vi "New Array.vi"(7 "prev index":i32, 8 "new index":i32, 9 "Array":T1[](array[typedef]), 10 "prev element":cluster{"X":dbl, "Y":dbl, "Z":dbl}, 11 "array":T2) -> (3 "array out":T2)   [LabVIEW 2014]
uses:
  Libraries/Map Data Folder/All-Lines.ctl
  Libraries/Map Data Folder/LineCluster.ctl
  Libraries/Map Data Folder/LineConnection.ctl
  Libraries/Contact Data/Position.ctl
  Libraries/Map Data Folder/Map Data.lvlib
  Libraries/Contact Data/Contact Data.lvlib
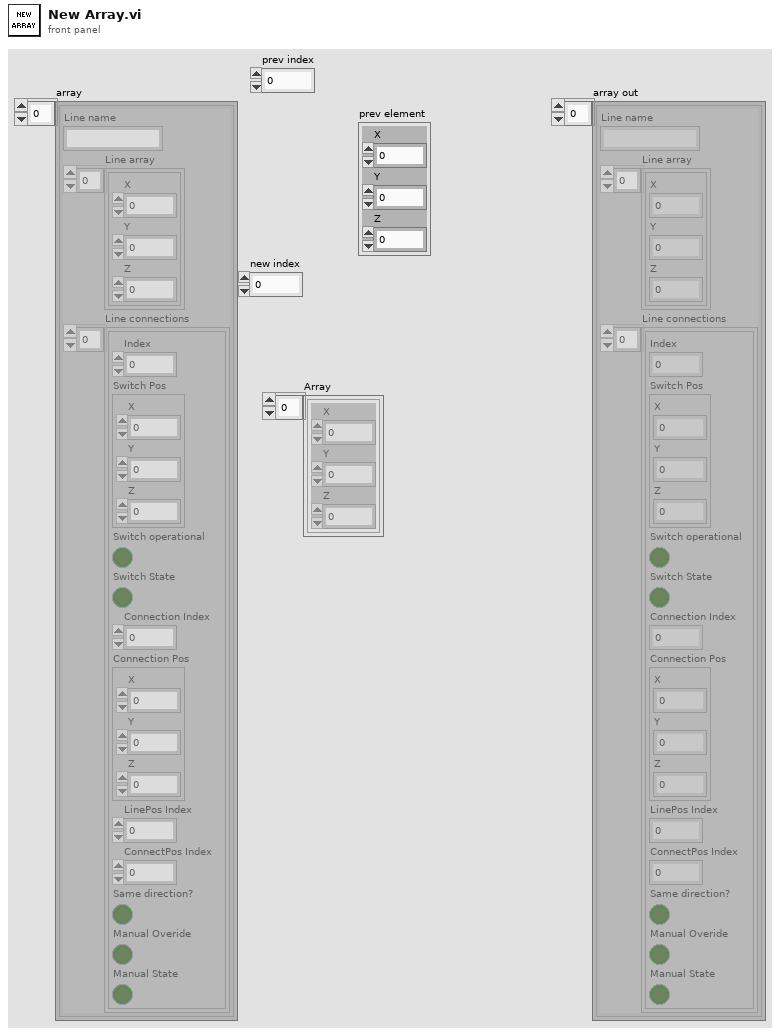
[diagram p1: front panel]
types:
  T1 = typedef "Contact Data.lvlib/Position.ctl" = cluster{"X":dbl, "Y":dbl, "Z":dbl}
  T2 = typedef "Map Data.lvlib/All-Lines.ctl" = T3[]
  T3 = typedef "Map Data.lvlib/LineCluster.ctl" = cluster{"Line name":string, "Line array":cluster{"X":dbl, "Y":dbl, "Z":dbl}[], "Line connections":T4[]}
  T4 = typedef "LineConnection.ctl" = cluster{"Index":i32, "Switch Pos":cluster{"X":dbl, "Y":dbl, "Z":dbl}, "Switch operational":bool, "Switch State":bool, "Connection Index":i32, "Connection Pos":cluster{"X":dbl, "Y":dbl, "Z":dbl}, "LinePos Index":i32, "ConnectPos Index":i32, "Same direction?":bool, "Manual Overide":bool, "Manual State":bool}
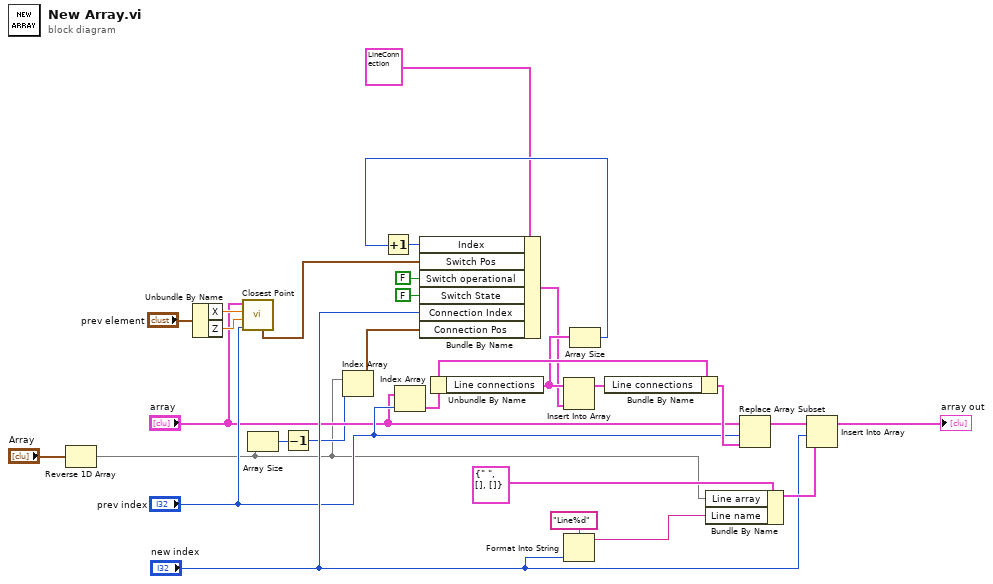
[diagram p0: block diagram]
diagram:
  n1 = Reverse 1D Array(array="Array") -> (reversed array=w3:T1[])
  n2 = Unbundle By Name("prev element") -> ("X"=w14:dbl, "Z"=w13:dbl)
  n3 = call "Closest Point.vi"("index"="prev index", "Y in"=w13, "X in"=w14, "All Lines"="array") -> ("element"=w8:cluster{"X":dbl, "Y":dbl, "Z":dbl})  [unwired: 5 in, 2 out]
  n4 = Array Size(array=w3) -> (size(s)=w6:i32)
  n5 = Decrement(x=w6) -> (x-1=w5:i32)
  n6 = Index Array(array=w3, index=w5) -> (element=w7:T1)
  n7 = Index Array(array="array", index="prev index") -> (element=w23:T3)
  n8 = Unbundle By Name(w23) -> ("Line connections"=w19:T4[])
  n9 = Format Into String(format string="Line%d", "new index") -> (resulting string=w25:string)  [unwired: 2 in, 1 out]
  n10 = Array Size(array=w19) -> (size(s)=w18:i32)
  n11 = Increment(x=w18) -> (x+1=w17:i32)
  n12 = Bundle By Name(cluster=T4 {"Index"=0, "Switch Pos"={"X"=0.0, "Y"=0.0, "Z"=0.0}, "Switch operational"=FALSE, "Switch State"=FALSE, "Connection Index"=0, "Connection Pos"={"X"=0.0, "Y"=0.0, "Z"=0.0}, "LinePos Index"=0, "ConnectPos Index"=0, "Same direction?"=FALSE, "Manual Overide"=FALSE, "Manual State"=FALSE}, "Index"=w17, "Switch Pos"=w8, "Switch operational"=FALSE, "Switch State"=FALSE, "Connection Index"="new index", "Connection Pos"=w7) -> (w2:T4)
  n13 = Insert Into Array(array=w19, new element=w2) -> (w22:T4[])  [unwired: 1 in]
  n14 = Bundle By Name(cluster=w23, "Line connections"=w22) -> (w21:T3)
  n15 = Bundle By Name(cluster=T3 {"Line name"=" ", "Line array"=[], "Line connections"=[]} ("Line Cluster 2"), "Line array"=w3, "Line name"=w25) -> (w28:T3)
  n16 = Replace Array Subset(array="array", new element=w21, index="prev index") -> (w20:T2)
  n17 = Insert Into Array(array=w20, index="new index", new element=w28) -> (→"array out":T2)
